vi "Error Query.vi"(0 "VISA resource name":refnum<visa-resource-name>, 5 "Input Read Buffer 1":string, 7 "Input Read Buffer 2":string, 11 "error in (no error)":errorcluster) -> (1 "Error Code 1":i32[](array[numeric]), 2 "Error Code 2":i32[](array[numeric]), 4 "VISA resource name out":refnum<visa-resource-name>, 8 "Error Message 1":string, 10 "Error Message 2":string, 15 "error out":errorcluster)   [LabVIEW 2019, in "BK Precision 178XB Series.lvlib"]
doc: "Queries the 85xx series DC load for any errors from a sent command frame. The instrument returns a 26 byte return command frame whenever a command sent to the instrument has errors. It is recommended that after each write operation, a read operation is done to capture the return command frame. This VI then takes the return command frame at the <b>Input Read Buffer</b> to extract and output the error code and error message. Up to 4 inputs (Input Read Buffer 1, 2, 3, 4) can be checked simultaneously (For driver VIs with multiple write operations) and their respective error codes (Error Code 1, 2, 3, 4) and error messages (Error Message 1, 2, 3, 4) will be at the output. Errors are also clustered together at <b>error out</b>.\n\nIf there is no string at any of the Input Read Buffers 1, 2, 3, and/or 4, no error messages will be returned.\n\nNote:\nThis VI is called automatically by most driver VIs so it is not usually necessary to call this in an application."
uses:
  BK Precision 178XB Series.lvlib
panel:
  # "(c) 2009 B&K PRECISION CORPORATION.  ALL RIGHTS RESERVED."
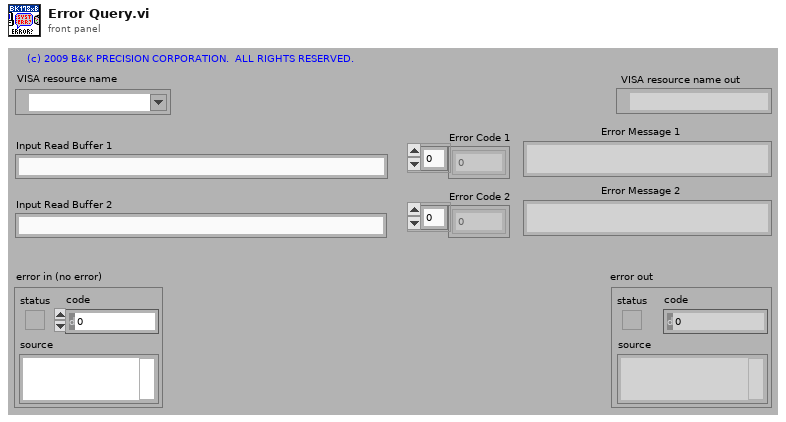
[diagram p1: front panel]
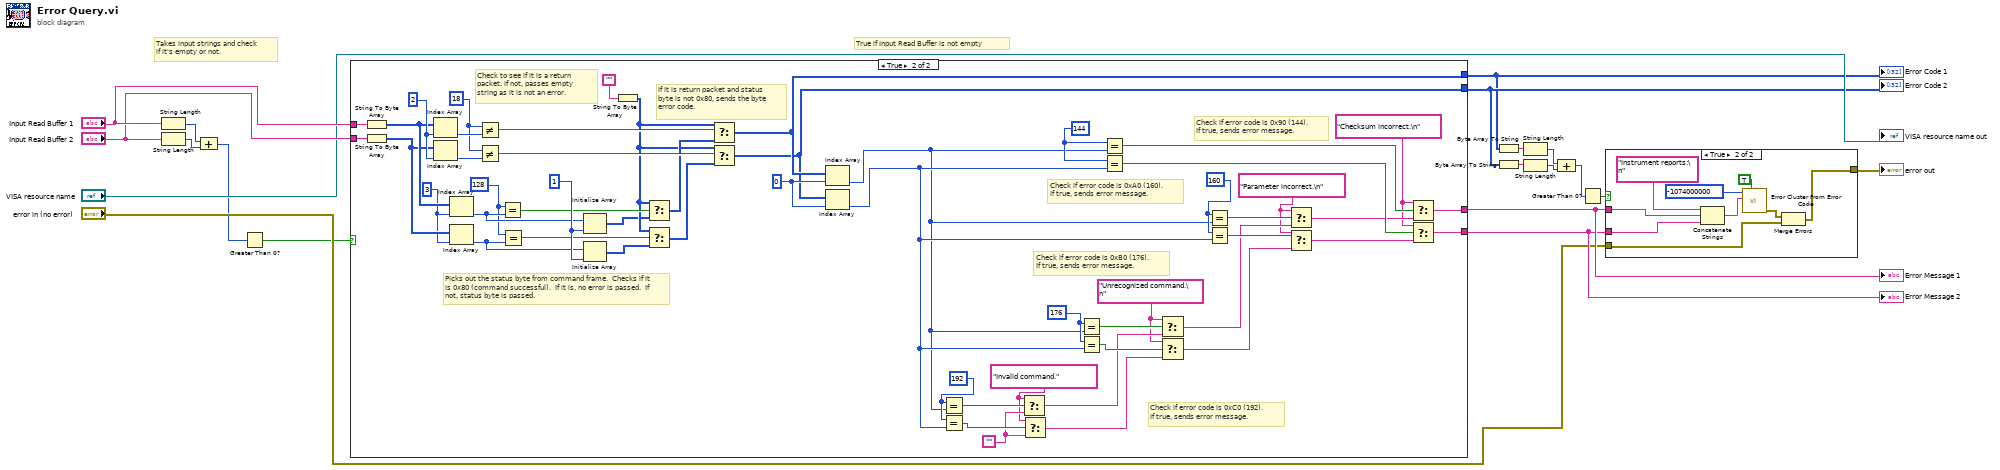
[diagram p0: block diagram]
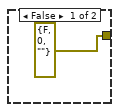
[diagram p2: hidden frame]
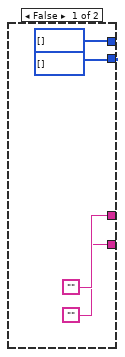
[diagram p3: hidden frame]
diagram:
  # "Takes input strings and check\nif it's empty or not."
  # "True if Input Read Buffer is not empty"
  n1 = String Length(string="Input Read Buffer 1") -> (length=w19:i32)
  n2 = String Length(string="Input Read Buffer 2") -> (length=w18:i32)
  n3 = Compound Arithmetic op=ADD(w19, w18) -> (w3:i32)
  n4 = Greater Than 0?(x=w3) -> (x > 0?=w2:bool)
  n5 = case shown="True" w2 {
    tunnel: "Input Read Buffer 1" -> [_ w76]
    tunnel: "Input Read Buffer 2" -> [_ w75]
    tunnel: [i32[] [] w40] -> w7
    tunnel: [i32[] [] w39] -> w8
    tunnel: ["" w42] -> w14
    tunnel: ["" w41] -> w13
    frame False {
    }
    frame True {
      w30 = u8 128
      w52 = ""
      w25 = "Invalid command." ("Source")
      w51 = u8 192
      w56 = u8 176
      w26 = "Unrecognized command.\n" ("Source")
      w27 = "Parameter incorrect.\n" ("Source")
      w60 = u8 160
      w24 = "Checksum incorrect.\n" ("Source")
      w63 = u8 144
      w64 = 0
      w66 = u8 1
      w67 = u8 3
      w71 = u8 18
      w74 = u8 2
      # "Picks out the status byte from command frame.  Checks if it is 0x80 (command successful).  If it is, no error is passed.  If not, status byte is passed."
      # "Check if error code is 0x90 (144).\nIf true, sends error message."
      # "Check if error code is 0xA0 (160).\nIf true, sends error message."
      # "Check if error code is 0xB0 (176).\nIf true, sends error message."
      # "Check if error code is 0xC0 (192).\nIf true, sends error message."
      # "If it is return packet and status\nbyte is not 0x80, sends the byte\nerror code."
      # "Check to see if it is a return packet. If not, passes empty string as it is not an error."
      n6 = String To Byte Array(string=w76) -> (unsigned byte array=w69:u8[])
      n7 = String To Byte Array(string=w75) -> (unsigned byte array=w68:u8[])
      n8 = Index Array(array=w69, index=w74) -> (element=w73:u8)
      n9 = Index Array(array=w68, index=w74) -> (element=w72:u8)
      n10 = Index Array(array=w69, index=w67) -> (element=w35:u8)
      n11 = Index Array(array=w68, index=w67) -> (element=w28:u8)
      n12 = Not Equal?(x=w71, y=w73) -> (x != y?=w38:bool)
      n13 = Not Equal?(x=w71, y=w72) -> (x != y?=w70:bool)
      n14 = Equal?(x=w30, y=w35) -> (x = y?=w37:bool)
      n15 = Equal?(x=w30, y=w28) -> (x = y?=w33:bool)
      n16 = Initialize Array(w35, w66) -> (w32:u8[])
      n17 = Initialize Array(w28, w66) -> (w31:u8[])
      n18 = String To Byte Array(string="") -> (unsigned byte array=w34:u8[])
      n19 = Select(t=w34, s=w37, f=w32) -> (s? t:f=w36:u8[])
      n20 = Select(t=w34, s=w33, f=w31) -> (s? t:f=w29:u8[])
      n21 = Select(t=w34, s=w38, f=w36) -> (s? t:f=w40:u8[])
      n22 = Select(t=w34, s=w70, f=w29) -> (s? t:f=w39:u8[])
      n23 = Index Array(array=w40, index=w64) -> (element=w49:u8)
      n24 = Index Array(array=w39, index=w64) -> (element=w50:u8)
      n25 = Equal?(x=w51, y=w49) -> (x = y?=w54:bool)
      n26 = Equal?(x=w51, y=w50) -> (x = y?=w53:bool)
      n27 = Select(t=w25, s=w54, f=w52) -> (s? t:f=w48:string)
      n28 = Select(t=w25, s=w53, f=w52) -> (s? t:f=w47:string)
      n29 = Equal?(x=w56, y=w49) -> (x = y?=w57:bool)
      n30 = Equal?(x=w56, y=w50) -> (x = y?=w55:bool)
      n31 = Equal?(x=w63, y=w49) -> (x = y?=w62:bool)
      n32 = Equal?(x=w63, y=w50) -> (x = y?=w61:bool)
      n33 = Select(t=w26, s=w57, f=w48) -> (s? t:f=w46:string)
      n34 = Select(t=w26, s=w55, f=w47) -> (s? t:f=w45:string)
      n35 = Equal?(x=w60, y=w49) -> (x = y?=w59:bool)
      n36 = Equal?(x=w60, y=w50) -> (x = y?=w58:bool)
      n37 = Select(t=w27, s=w59, f=w46) -> (s? t:f=w44:string)
      n38 = Select(t=w27, s=w58, f=w45) -> (s? t:f=w43:string)
      n39 = Select(t=w24, s=w62, f=w44) -> (s? t:f=w42:string)
      n40 = Select(t=w24, s=w61, f=w43) -> (s? t:f=w41:string)
    }
  }
  "Error Message 1" <- w14
  "Error Code 1" <- w7
  "Error Code 2" <- w8
  "Error Message 2" <- w13
  n41 = Byte Array To String(unsigned byte array=w7) -> (string=w10:string)
  n42 = Byte Array To String(unsigned byte array=w8) -> (string=w9:string)
  n43 = String Length(string=w10) -> (length=w6:i32)
  n44 = String Length(string=w9) -> (length=w5:i32)
  n45 = Compound Arithmetic op=ADD(w6, w5) -> (w4:i32)
  n46 = Greater Than 0?(x=w4) -> (x > 0?=w1:bool)
  n47 = case shown="True" w1 {
    tunnel: w14 -> [_ w81]
    tunnel: w13 -> [_ w80]
    tunnel: "error in (no error)" -> [_ w79]
    tunnel: [errorcluster {"status"=FALSE, "code"=0, "source"=""} ("error out") w78] -> w11
    frame False {
    }
    frame True {
      n48 = Concatenate Strings("Instrument reports:\n" ("Source"), w81, w80) -> (w83:string)
      n49 = call <vilib>:"Error Cluster From Error Code.vi"("show call chain? (False)"=TRUE, "error message (\"\")"=w83, "error code (0)"=-1074000000 ("Code")) -> ("error out"=w82:errorcluster)  [unwired: 6 in]
      n50 = Merge Errors(w82, w79) -> (w78:errorcluster)
    }
  }
  "error out" <- w11
  "VISA resource name out" <- "VISA resource name"
